vi "Collect Control References.vi"(8 "error in (no error)":errorcluster, 11 "Engine in":refnum<class "Engine.lvclass">) -> (0 "error out":errorcluster, 2 "Control References":T1(array[cluster]), 3 "Engine out":refnum<class "Engine.lvclass">)   [LabVIEW 2023, in "Engine.lvlib" / "Engine.lvclass"]
uses:
  Library/Engine.lvclass
  Library/Engine.lvclass/Engine.ctl
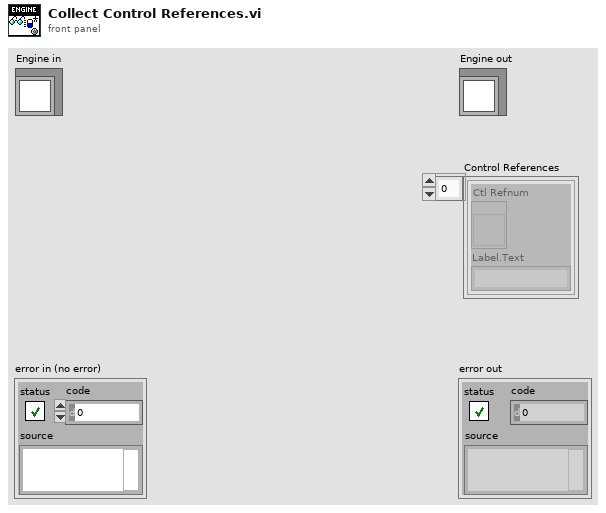
[diagram p1: front panel]
types:
  T1 = cluster{"Ctl Refnum":refnum<vi>, "Label.Text":string}[]
  T2 = typedef "Engine.lvlib/Engine.lvclass/Control Reference.ctl" = cluster{"Reference":refnum<vi>, "Label":string}
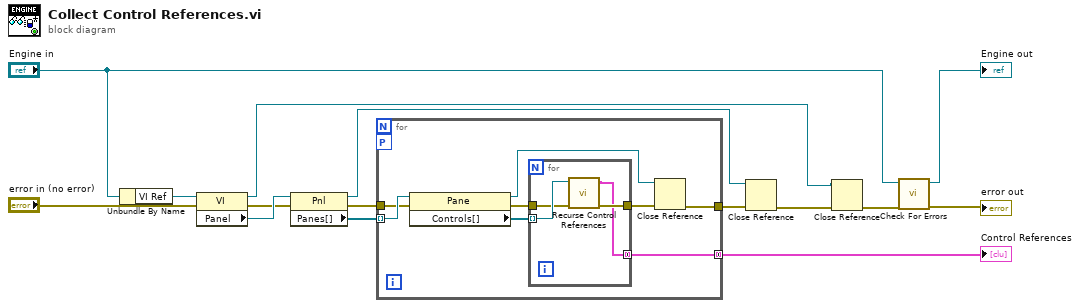
[diagram p0: block diagram]
diagram:
  n1 = Unbundle By Name("Engine in") -> ("VI Ref"=w15:refnum<vi>)
  n2 = property on="Property Node" class="VI"(reference=w15, error in="error in (no error)") -> (reference out=w8:refnum<vi>, error out=w2:errorcluster, "Panel"=w14:refnum<vi>)
  n3 = property on="Property Node" class="Pnl"(reference=w14, error in=w2) -> (reference out=w10:refnum<vi>, error out=w12:errorcluster, "Panes[]"=w13:refnum<vi>[])
  n4 = for {
    tunnel: w13 -> [w23] mode=indexing
    tunnel: [w19] -> w11
    tunnel: w12 -> [w18]
    workers-P: _ -> [_]
    tunnel: [w16] -> w1 mode=concatenating
    n5 = property on="Property Node" class="Pane"(reference=w23, error in=w18) -> (reference out=w17:refnum<vi>, error out=w21:errorcluster, "Controls[]"=w22:refnum<vi>[])
    n6 = for {
      tunnel: w22 -> [w27] mode=indexing
      tunnel: w21 -> [w26]
      tunnel: [w25] -> w20
      tunnel: [w24] -> w16 mode=concatenating
      n7 = call "Recurse Control References.vi"("error in (no error)"=w26, "Ctl Refnum"=w27) -> ("error out"=w25:errorcluster, "Control References"=w24:T2[])  [unwired: 8 in]
    }
    n8 = Close Reference(reference=w17, error in (no error)=w20) -> (error out=w19:errorcluster)
  }
  "Control References" <- w1
  n9 = Close Reference(reference=w10, error in (no error)=w11) -> (error out=w9:errorcluster)
  n10 = Close Reference(reference=w8, error in (no error)=w9) -> (error out=w7:errorcluster)
  n11 = call "Check For Errors.vi"("error in"=w7, "Engine in"="Engine in") -> ("error out"=→"error out":errorcluster, "Engine out"=→"Engine out":refnum<class "Engine.lvclass">)  [unwired: 8 in]
